vi "Driver Controller Inputs.vi"() -> ()   [LabVIEW 2017]
panel:
  in  "Driver Controller":string
  out "Button 10":bool
  out "Button 9":bool
  out "Button 8":bool
  out "Button 7":bool
  out "Button 6":bool
  out "Button 5":bool
  out "Button 4":bool
  out "Button 3":bool
  out "Button 2":bool
  out "Button 1":bool
  out "Button 0":bool
  in  "Axes 10":dbl
  in  "Axes 9":dbl
  in  "Axes 8":dbl
  in  "Axes 7":dbl
  in  "Axes 6":dbl
  in  "Axes 5":dbl
  in  "Axes 4":dbl
  in  "Axes 3":dbl
  in  "Axes 2":dbl
  in  "Axes 1":dbl
  in  "Axes 0":dbl
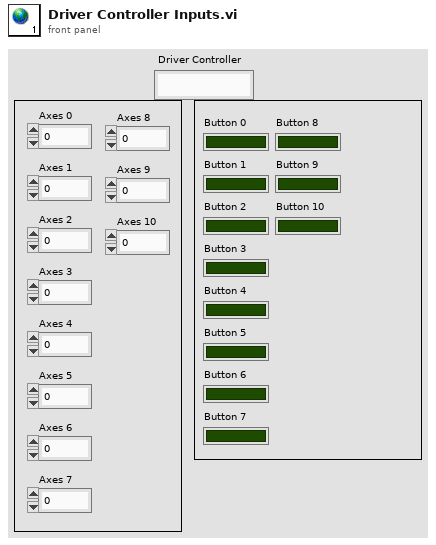
[diagram p1: front panel]
diagram:
